vi "Is GUI Running (library variable).vi"() -> ()   [LabVIEW 2023, in "Error Manager.lvlib" / "New Error Dialogue GUI.lvlib"]
uses:
  New Error Dialogue GUI.lvlib
panel:
  out "Is GUI Running?":bool
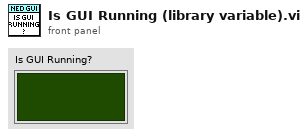
[diagram p1: front panel]
diagram:
